vi "Control_Variable de Estados_Diagrama.vi"() -> ()   [LabVIEW 2020]
uses:
  <vilib>/Simulation/Scripting/Companion Diagram/SimConfigNode/SimParams.ctl
  <vilib>/Simulation/Scripting/Companion Diagram/SimConfigNode/_simSolvers.ctl
  <vilib>/Simulation/Implementation/Shared/SIMSCR Execution Mode.ctl
  <vilib>/Simulation/Param Hierarchy/Typedefs/SIMPH Param Control Actions.ctl
  <vilib>/Simulation/Implementation/Shared/NILVSim_ParamChanged.vi
  <vilib>/Simulation/Implementation/Shared/NILVSIM_BeginStep.vi
  <vilib>/Simulation/Utility/Implementation/SIM Halt.vi
  <vilib>/Simulation/DataSources/Implementation/NILVSim Pulse Generator.llb/SIM Pulse Generator (scalar).vi
  <vilib>/Simulation/ContinuousLinear/Implementation/NILVSim State Space.llb/SIM State Space Distributor (SISO).vi
  <vilib>/Simulation/SignalArithmetic/Implementation/NILVSim Gain.llb/SIM Gain (scalar).vi
  <vilib>/Simulation/SignalDisplay/Implementation/NILVSim Time Waveform.llb/SIM Time Waveform (vector).vi
  <vilib>/Simulation/ContinuousLinear/Implementation/NILVSim State Space.llb/SIM State Space Collector (SISO).vi
  <vilib>/Simulation/Implementation/Shared/NILVSim_Manager.vi
  <vilib>/Utility/error.llb/Clear Errors.vi
  <vilib>/Simulation/Implementation/Shared/NILVSim_FinalizeModel.vi
  <vilib>/Simulation/DiscreteLinear/Implementation/NILVSim Discrete Transfer Function Buffered.llb/SIM Discrete Transfer Function Distributor (MIMO).vi
  <vilib>/Simulation/ContinuousLinear/Implementation/NILVSim Transfer Function.llb/SIM Transfer Function Collector (MIMO).vi
  <vilib>/Simulation/DataSources/Implementation/NILVSim Step.llb/SIM Step (scalar).vi
  <vilib>/Simulation/Implementation/Shared/SIM Unbundle Sim Info.vi
  <vilib>/Simulation/Implementation/Shared/NILVSim_Initialize.vi
  <vilib>/Simulation/Utility/Implementation/NILVSim Get Time and IsAcceptedStep.vi
  <vilib>/Simulation/Implementation/Shared/SIMSH Read Queue.vi
  <vilib>/Simulation/Implementation/Shared/NILVSim_GetModelError.vi
  <vilib>/Simulation/Implementation/Shared/SIM Bundle Sim Info.vi
  <vilib>/Simulation/Scripting/Companion Diagram/SimConfigNode/SimDog.xnode
  <vilib>/Simulation/Implementation/XNodeFramework/SimXNode/SimX.xnode
  <vilib>/Simulation/Implementation/Shared/NI_SIM_Implementation.lvlib
  <vilib>/Simulation/DiscreteLinear/Implementation/NILVSim Discrete Transfer Function Buffered.llb/SIM Discrete Transfer Function Buffered (MIMO).vi
  <vilib>/Simulation/ContinuousLinear/Implementation/NILVSim State Space.llb/SIM State Space (SISO).vi
panel:
  out "9)":waveform(dbl)[](graph)
  in  "STOP 4":bool
  out "9) Respuesra del sistema con funcion cuadratica":waveform(dbl)[](graph)
  in  "STOP 3":bool
  out "2) Respuesta de la planta con escalon unitario":waveform(dbl)[](graph)
  in  "STOP 2":bool
  in  "STOP":bool
  out "2)":waveform(dbl)[](graph)
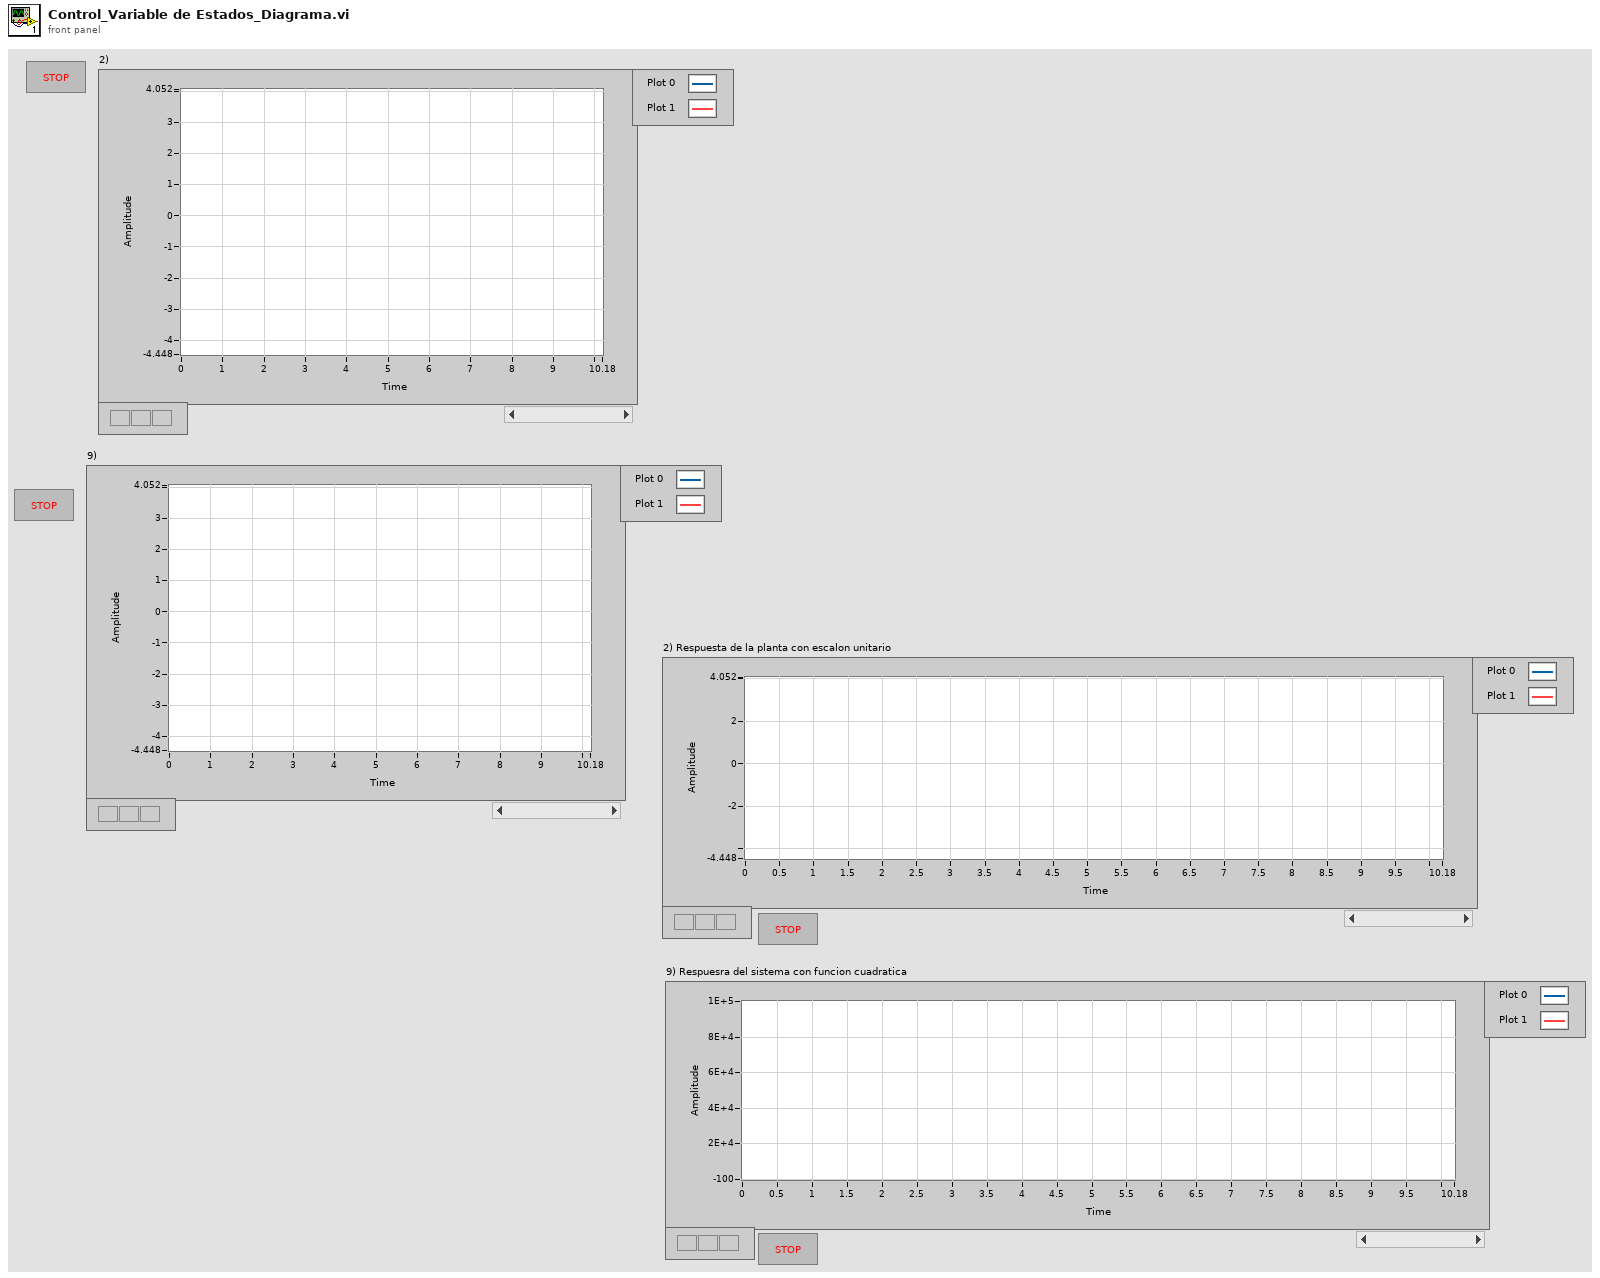
[diagram p1: front panel]
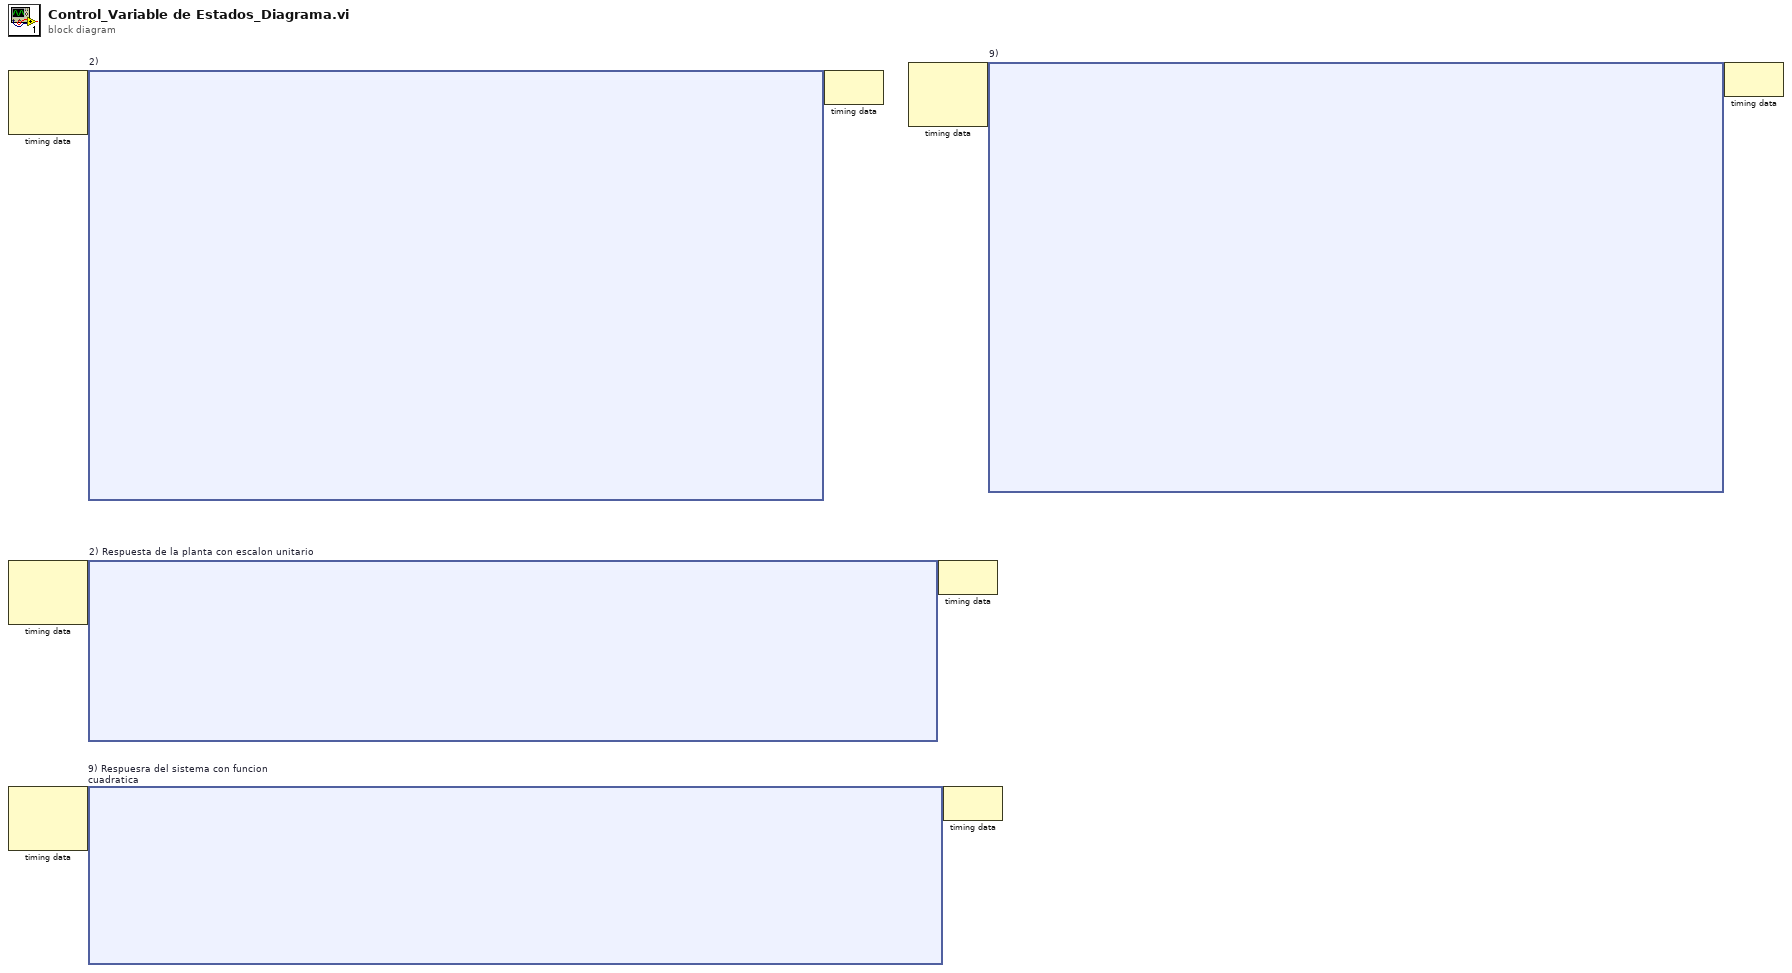
[diagram p0: block diagram]
diagram:
  n1 = node-c288() -> (w8:variant)  [unwired: 3 in]
  n2 = node-c288() -> (w6:variant)  [unwired: 3 in]
  n3 = node-c288() -> (w4:variant)  [unwired: 3 in]
  n4 = node-c254 "2)"(w8) -> (w7:variant)
  n5 = node-c254 "2) Respuesta de la planta con escalon unitario"(w6) -> (w5:variant)
  n6 = node-c254 "9) Respuesra del sistema con funcion cuadratica"(w4) -> (w3:variant)
  n7 = node-c288(w7) -> ()  [unwired: 1 out]
  n8 = node-c288() -> (w2:variant)  [unwired: 3 in]
  n9 = node-c288(w5) -> ()  [unwired: 1 out]
  n10 = node-c288(w3) -> ()  [unwired: 1 out]
  n11 = node-c254 "9)"(w2) -> (w1:variant)
  n12 = node-c288(w1) -> ()  [unwired: 1 out]
